vi "PmuAnalysis.vi"() -> ()   [LabVIEW 2018, in "Visualization.lvlib" / "VisualizeAnalysis.lvclass"]
uses:
  VisualizeAnalysis.lvclass
  VisualizeBase/VisualizeBase_class/SubVIs/VisualizationOptions.ctl
  <vilib>/Utility/miscctls.llb/LVRectTypeDef.ctl
  <vilib>/event_ctls.llb/usereventprio.ctl
  VisualizeBase/VisualizeBase_class/Requests/VisUserEventType.ctl
  <extravilib>/ChannelInstances/Tag-bool/Write With Abort.vi
  <extravilib>/ChannelInstances/Tag-bool/Read With Abort.vi
  <extravilib>/ChannelInstances/Tag-bool/Instantiate.vi
  <vilib>/Utility/error.llb/Error Cluster From Error Code.vi
  <extravilib>/ChannelInstances/Tag-bool/Endpoint.vi
  <vilib>/Utility/file.llb/Read From Spreadsheet File (DBL).vi
  <extravilib>/ChannelInstances/Tag-bool/EndpointRead.vi
  <vilib>/ErrorRing/Error Ring.xnode
  <userlib>/NIST/NISTErrorLib/NISTErrorLib.lvlib
  VisualizeBase/VisualizeBase_class/VisualizeBase.lvclass
  Analysis/AnalysisModule/AnalysisModule.lvlib
  Visualization.lvlib
  Sensor/VisualizeSensor.lvclass
  <extravilib>/ChannelInstances/Tag-bool.lvlib
  TestClass/Test.lvclass
  StatusAndLog/VisualizeStatus.lvclass
panel:
  in  "INIFilePath":path
  out "VisualizationProperties":T1={"PauseAtStartup"=TRUE, "LogData"=FALSE, "LaunchInSubPanel"=TRUE, "FPMonitor"=0, "FPWindowBounds"={"Left"=0, "Top"=0, "Right"=0, "Bottom"=0}, "MonitorBounds"={"Left"=0, "Top"=0, "Right"=0, "Bottom"=0}}
  in  "ModuleID":i32
  in  "btnClearTest":bool
  in  "btnReset":bool
  in  "btnPause":bool
  in  "btnOpen":bool
  in  "btnStop":bool
  in  "PluginName":string="Sensor.RoomAlert1"
  in  "Log Data":bool=TRUE
  out "Data from file":dbl[][](array[numeric])
  out "TVE":cluster{timestamp[], dbl[]}[](graph)
  out "FE":dbl(graph)=1.1347977483922023e-05
  out "ErrorArray":errorcluster[](array[cluster])
  out "RFE":dbl(graph)=-0.0019269131938461162
  out "Data real time":dbl[](array[numeric])
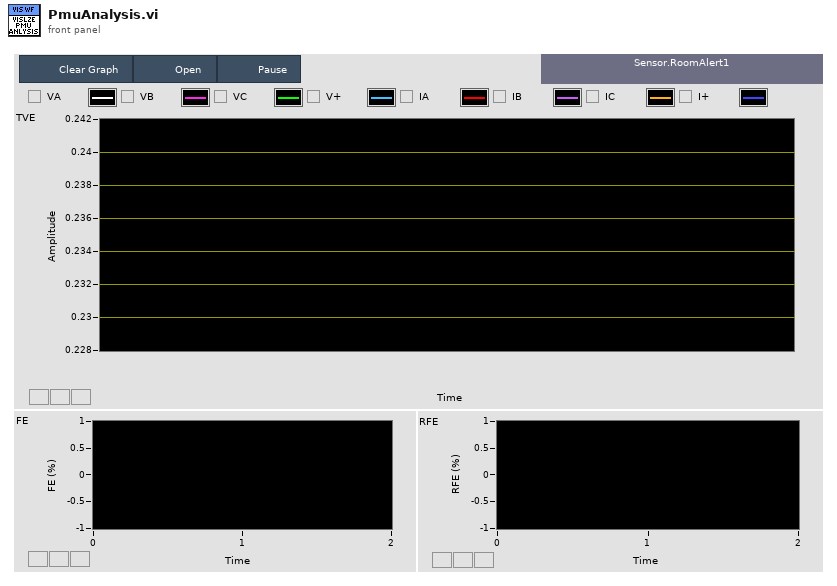
[diagram p1: front panel]
types:
  T1 = typedef "Visualization.lvlib/VisualizeBase.lvclass/VisualizationOptions.ctl" = cluster{"PauseAtStartup":bool, "LogData":bool, "LaunchInSubPanel":bool, "FPMonitor":u16, "FPWindowBounds":T2, "MonitorBounds":cluster{"Left":i16, "Top":i16, "Right":i16, "Bottom":i16}}
  T2 = typedef "LVRectTypeDef.ctl" = cluster{"Left":i16, "Top":i16, "Right":i16, "Bottom":i16}
  T3 = typedef "Visualization.lvlib/VisualizeBase.lvclass/VisRequestEvents.ctl" = cluster{"StopRequest":refnum<user-event>, "ResetRequest":refnum<user-event>, "FP Pop In or Out":refnum<user-event>}
  T4 = typedef "AnalysisModule.lvlib/clBroadcastEvents.ctl" = cluster{"DidInit":refnum<user-event>, "StatusUpdate":refnum<user-event>, "ErrorReport":refnum<user-event>, "DidStop":refnum<user-event>, "PathToINI":refnum<user-event>, "Config":refnum<user-event>, "ResultReport":refnum<user-event>, "FunctionClass":refnum<user-event>, "State":refnum<user-event>, "FunctionParams":refnum<user-event>, "Duration":refnum<user-event>}
  T5 = enum16{"open", "open or create", "create or replace", "create", "open (read-only)"}
  T6 = typedef "Visualization.lvlib/VisualizeBase.lvclass/VisUserEventType.ctl" = cluster{"BusIndex":i8, "Data":variant}
  T7 = typedef "usereventprio.ctl" = enum32{"high priority", "normal priority"}
  T8 = typedef "Tag-bool.lvlib/))Channel.ctl" = refnum<queue>
  T9 = typedef "sizeaction.ctl" = enum32{"Minimized", "Maximized", "Resized"}
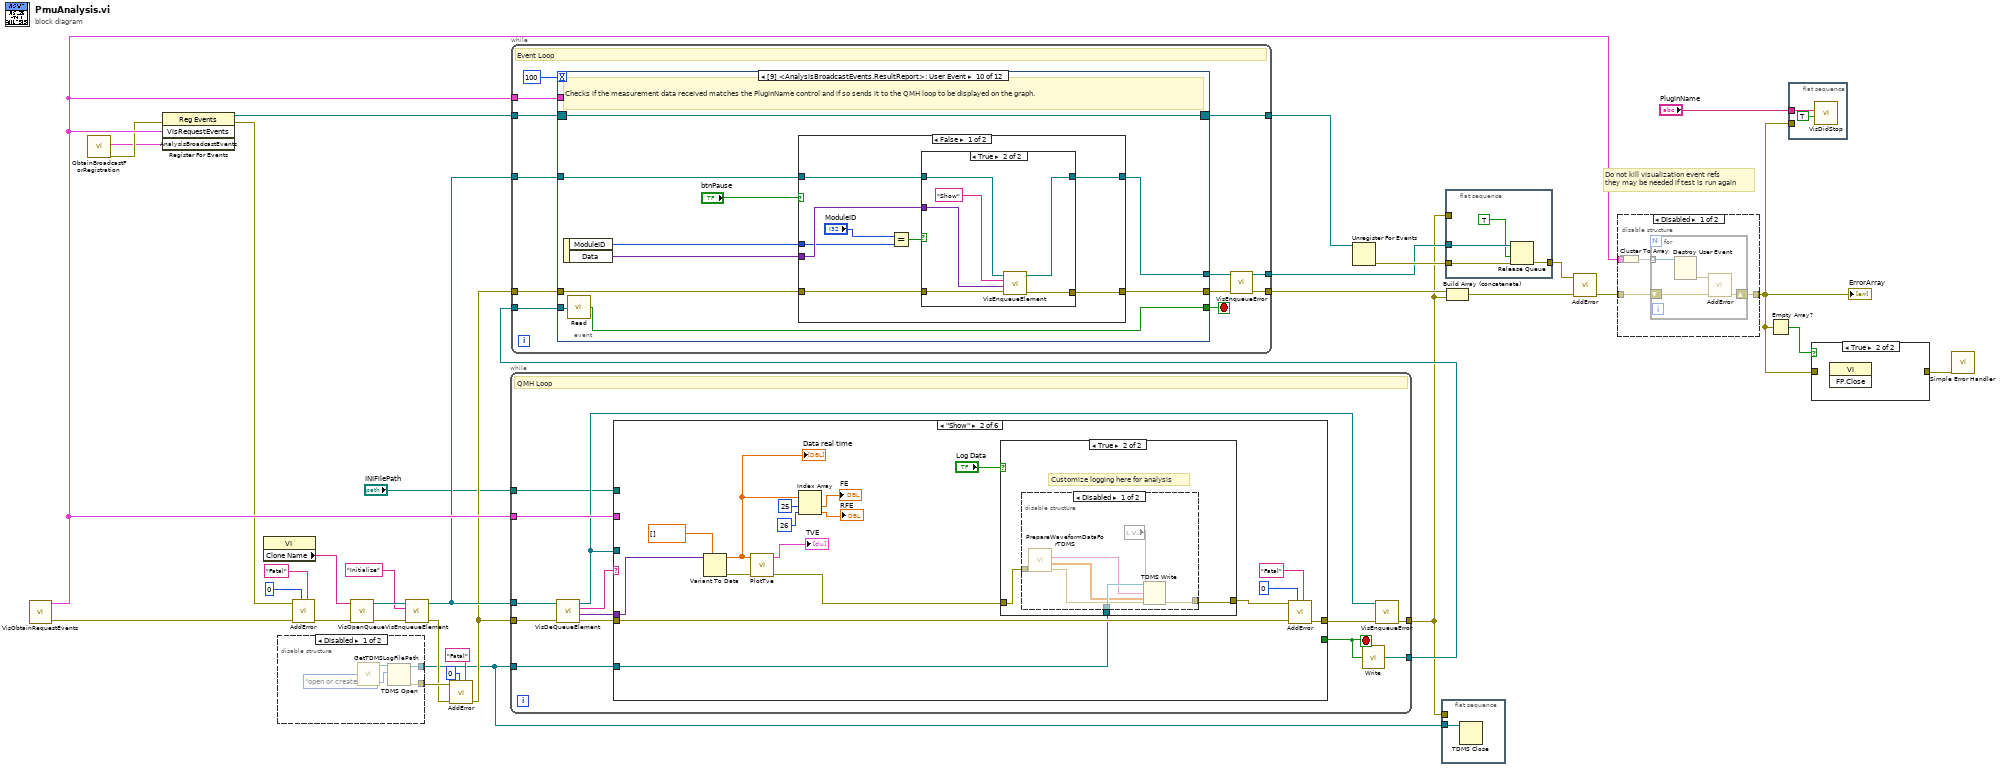
[diagram p0: block diagram]
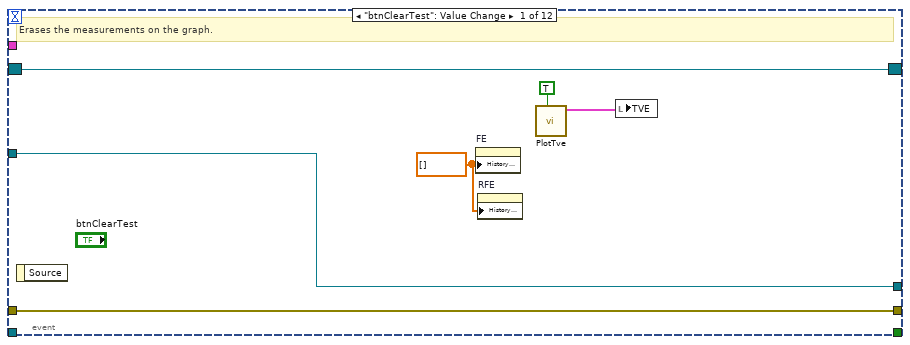
[diagram p4: hidden frame]
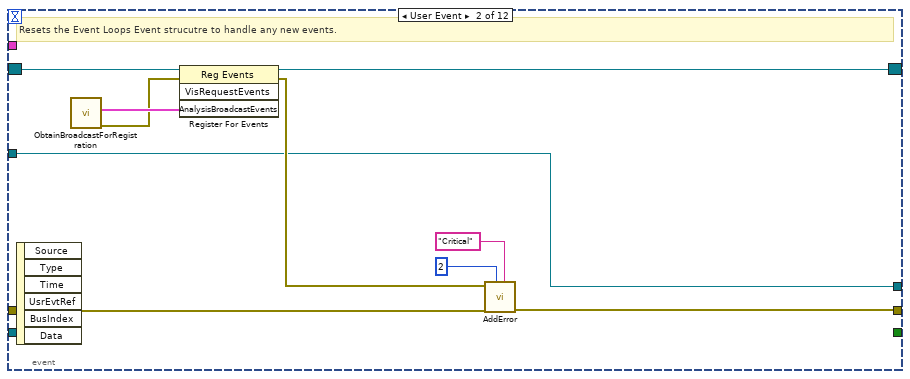
[diagram p5: hidden frame]
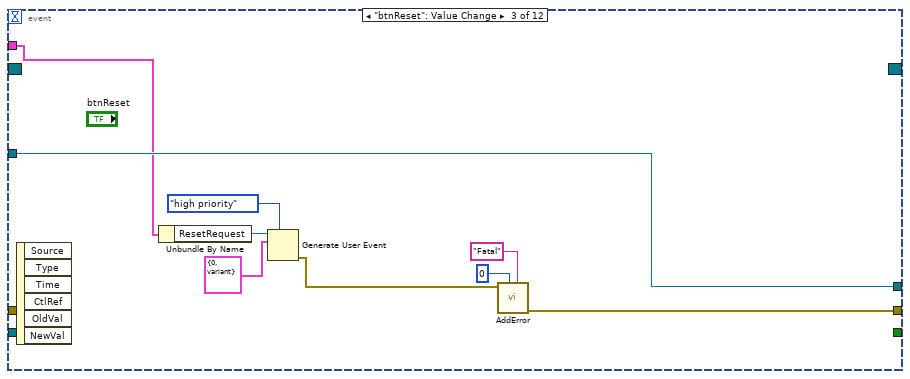
[diagram p6: hidden frame]
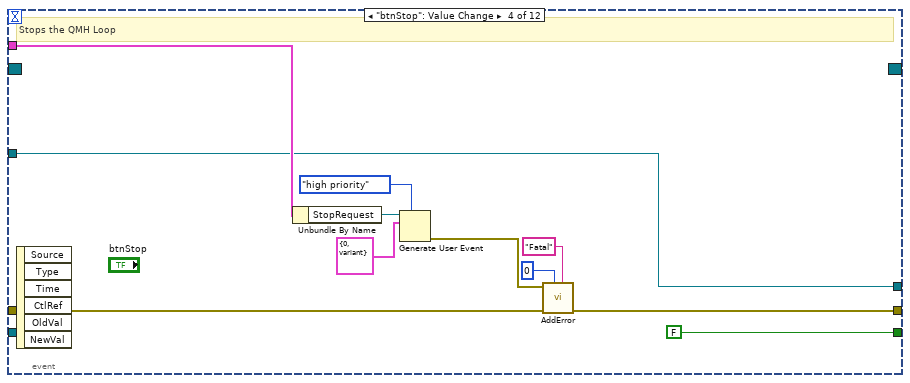
[diagram p7: hidden frame]
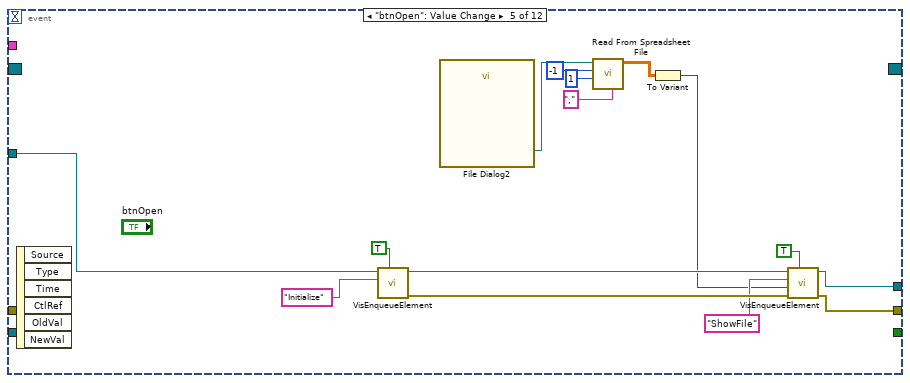
[diagram p8: hidden frame]
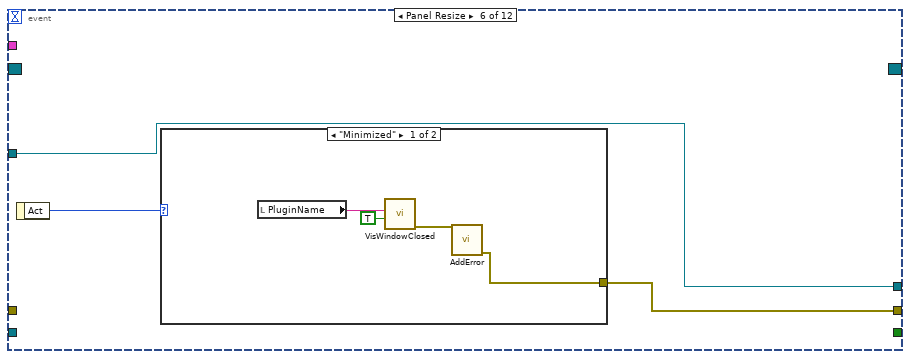
[diagram p9: hidden frame]
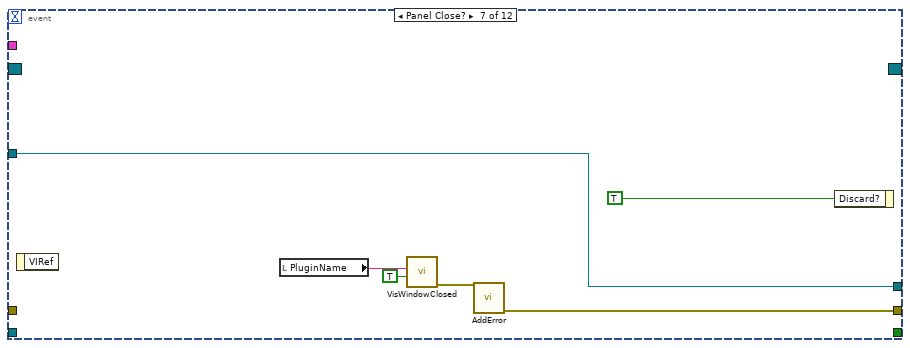
[diagram p11: hidden frame]
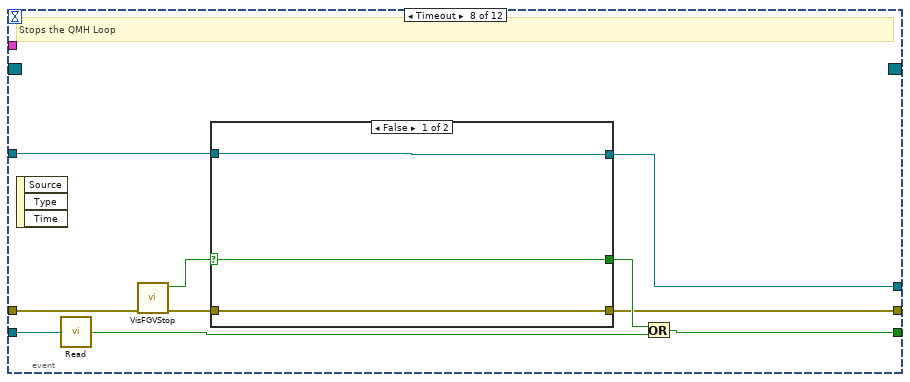
[diagram p12: hidden frame]
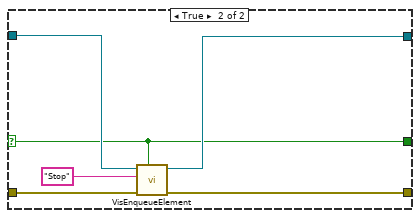
[diagram p13: hidden frame]
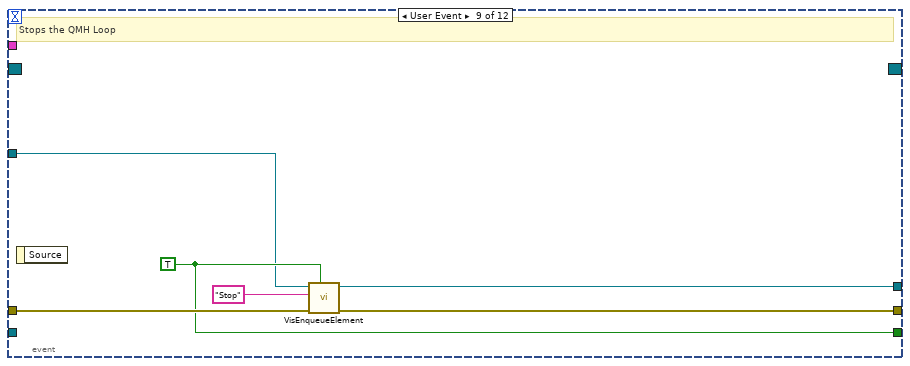
[diagram p14: hidden frame]
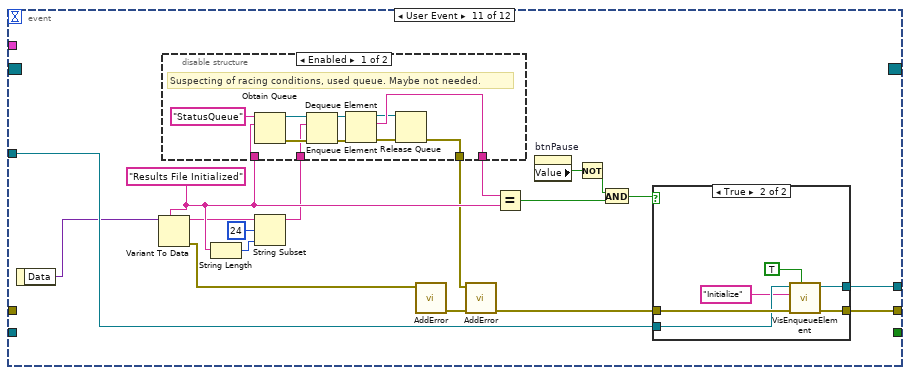
[diagram p17: hidden frame]
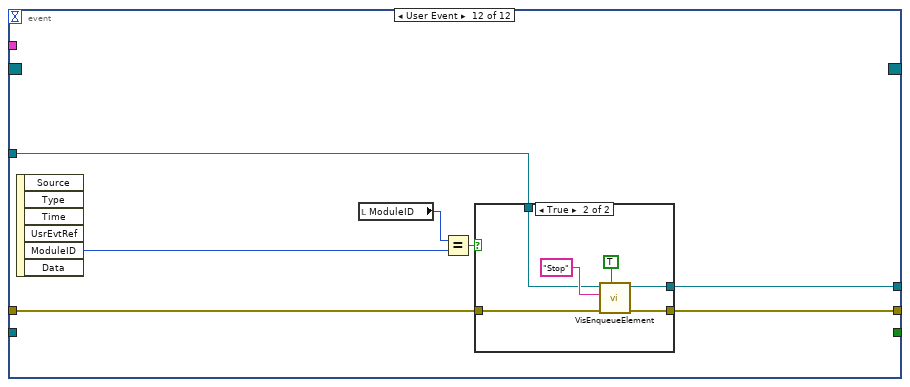
[diagram p20: hidden frame]
diagram:
  # "Do not kill visualization event refs\nthey may be needed if test is run again"
  n1 = call "VisObtainRequestEvents.vi"() -> ("Error"=w25:errorcluster[], "VisRequestEvents"=w27:T3)  [unwired: 10 in]
  n2 = call "ObtainBroadcastForRegistration.vi"() -> ("error out"=w5:errorcluster, "AnalysisBroadcastEvents"=w4:T4)  [unwired: 10 in]
  n3 = register-events(error in=w5, w27, w4) -> (reference out=w34:refnum<event-registration>, error out=w24:errorcluster)  [unwired: 1 in]
  n4 = property class="VI"() -> ("Clone Name"=w13:string)  [unwired: 2 in, 2 out]
  n5 = disable-structure shown="Disabled" {
    disable-tunnel: [w37 _] -> w10
    disable-tunnel: [w35 _] -> w7
    frame Disabled {
      n6 = call "GetTDMSLogFilePath.vi"() -> ("TDMS Log File Path"=w38:path)  [unwired: 11 in]
      n7 = TDMS Open(10:T5."open or create" ("operation (0:open)"), 11:w38) -> (0:w37:errorcluster, 3:w35:refnum<k34>)  [unwired: 5 in]
    }
    frame Enabled {
    }
  }
  n8 = call <userlib>:"AddError.vi"("Severity"="Fatal", "Priority"=u8 0, "ErrorArray In"=w25, "error in (no error)"=w24) -> ("ErrorArray Out"=w21:errorcluster[])  [unwired: 6 in, 1 out]
  n9 = call "VisOpenQueue.vi"("Error Array In"=w21, "QueueName"=w13) -> ("Error Array Out"=w19:errorcluster[], "queue out"=w20:refnum<queue>)  [unwired: 8 in]
  n10 = call "VisEnqueueElement.vi"("Error Array In"=w19, "Message"="Initialize", "queue in"=w20) -> ("Error Array Out"=w9:errorcluster[], "queue out"=w17:refnum<queue>)  [unwired: 7 in]
  n11 = call <userlib>:"AddError.vi"("Severity"="Fatal", "Priority"=u8 0, "ErrorArray In"=w9, "error in (no error)"=w10) -> ("ErrorArray Out"=w8:errorcluster[])  [unwired: 6 in, 1 out]
  n12 = while {
    tunnel: w8 -> [w45]
    tunnel: [w48] -> w6
    tunnel: w17 -> [w44]
    tunnel: w27 -> [w50]
    tunnel: [w41] -> w14
    tunnel: w7 -> [w40]
    tunnel: "INIFilePath" -> [w39]
    stop <- w51 stop-if-true
    # "QMH Loop"
    n13 = call "VisDeQueueElement.vi"("Error Array In"=w45, "Queue In"=w44) -> ("Error Array Out"=w43:errorcluster[], "Data"=w46:variant, "Message"=w47:string, "Queue Out"=w42:refnum<queue>)  [unwired: 6 in]
    n14 = case shown="\"Show\"" w47 {
      selector: w47 -> [_ _ _ w114 _ _]
      tunnel: w46 -> [_ w63 w89 _ w133 _]
      tunnel: w43 -> [w55 w76 _ w112 _ w162]
      tunnel: [w54 w77 _ w111 w123 w161] -> w49
      tunnel: [_ _ _ _ w129 TRUE] -> w51
      tunnel: w50 -> [_ _ _ _ w128 _]
      tunnel: w42 -> [_ _ _ _ w127 _]
      tunnel: w40 -> [_ w71 _ _ _ _]
      tunnel: w39 -> [w53 _ _ _ _ w160]
      frame "Initialize" {
        w60 = dbl[] [] ("History Data")
        (unwired) dbl[][] [] ("History Data")
        n15 = call "ApplyVisOptions.vi"("INIFilePath"=w53) -> ("error out"=w56:errorcluster, "VisualizationProperties"=→"VisualizationProperties":T1)  [unwired: 9 in]
        n16 = call <userlib>:"AddError.vi"("Severity"="Inform", "ErrorArray In"=w55, "error in (no error)"=w56) -> ("ErrorArray Out"=w54:errorcluster[])  [unwired: 7 in, 1 out]
        n17 = property on="FE" class="WFChart (strict)"("History Data"=w60) -> ()  [unwired: 2 in, 2 out]
        n18 = property on="RFE" class="WFChart (strict)"("History Data"=w60) -> ()  [unwired: 2 in, 2 out]
        n19 = call "PlotTve.vi"("Clear? (f)"=TRUE) -> ("TVE"=w58:cluster{timestamp[], dbl[]}[])  [unwired: 9 in, 1 out]
        n20 = property on="TVE" class="XYGraph (strict)"("Value"=w58) -> ()  [unwired: 2 in, 2 out]
      }
      frame "Show" {
        n21 = Variant To Data(type=dbl[] [], Variant=w63) -> (data=w68:dbl[], error out=w61:errorcluster)  [unwired: 1 in]
        "Data real time" <- w68
        n22 = call "PlotTve.vi"("error in (no error)"=w61, "Data real time"=w68) -> ("error out"=w62:errorcluster, "TVE"=→"TVE":cluster{timestamp[], dbl[]}[])  [unwired: 8 in]
        n23 = Index Array(array=w68, index #1=25 ("index"), index #2=26 ("index")) -> (element #1=→"FE":dbl, element #2=→"RFE":dbl)
        n24 = case shown="True" "Log Data" {
          tunnel: w62 -> [w78 w80]
          tunnel: [w78 w81] -> w73
          tunnel: w71 -> [_ w79]
          frame False {
          }
          frame True {
            # "Customize logging here for analysis"
            n25 = disable-structure shown="Disabled" {
              disable-tunnel: [w88 _] -> w81
              disable-tunnel: w80 -> [w87 _]
              disable-tunnel: w79 -> [w85 _]
              frame Disabled {
                n26 = call "PrepareWaveformDataForTDMS.vi"("error in (no error)"=w87) -> ("error out"=w84:errorcluster, "Measurement Data"=w82:dbl[][], "Channel Names"=w83:string[])  [unwired: 8 in]
                n27 = local read item#-1() -> (w86)
                n28 = TDMS Write(0:w85, 5:w86, 7:w83, 9:w82, 11:w84) -> (15:w88:errorcluster)  [unwired: 1 in, 3 out]
              }
              frame Enabled {
              }
            }
          }
        }
        n29 = call <userlib>:"AddError.vi"("Severity"="Fatal" ("String"), "Priority"=u8 0, "ErrorArray In"=w76, "error in (no error)"=w73) -> ("ErrorArray Out"=w77:errorcluster[])  [unwired: 6 in, 1 out]
      }
      frame "ShowFile" {
        n30 = Variant To Data(type=dbl[][] [], Variant=w89) -> (data=w102:dbl[][])  [unwired: 1 in, 1 out]
        "Data from file" <- w102
        n31 = Index Array(array=w102, index (col) #1=1 ("disabled index (col)"), index (col) #2=4 ("index (col)"), index (col) #3=7 ("index (col)"), index (col) #4=10 ("index (col)")) -> (element #1=w98:dbl[], element #2=w99:dbl[], element #3=w100:dbl[], element #4=w105:dbl[])  [unwired: 4 in]
        n32 = Index Array(array=w102, index (col) #1=25 ("disabled index (col)"), index (col) #2=26 ("index (col)")) -> (element #1=w103:dbl[], element #2=w104:dbl[])  [unwired: 2 in]
        n33 = Array Size(array=w105) -> (size(s)=w106:i32)
        n34 = Initialize Array(1.0 ("element"), w106) -> (w107:dbl[])
        n35 = property on="FE" class="WFChart (strict)"("History Data"=w103) -> ()  [unwired: 2 in, 2 out]
        n36 = Build Array(w98, w99, w100, w105, w107) -> (w101:dbl[][])
        n37 = property on="RFE" class="WFChart (strict)"("History Data"=w104) -> ()  [unwired: 2 in, 2 out]
        n38 = Transpose 2D Array(2D array=w101) -> ()  [unwired: 1 out]
      }
      frame Default {
        n39 = xnode "Error Ring"("parameter 0"=w114) -> ("error out"=w113:errorcluster)
        n40 = call <userlib>:"AddError.vi"("Severity"="Inform" ("String"), "Priority"=u8 5, "ErrorArray In"=w112, "error in (no error)"=w113) -> ("ErrorArray Out"=w111:errorcluster[], "error out"=w110:errorcluster)  [unwired: 6 in]
        n41 = call <vilib>:"Clear Errors.vi"("error in (no error)"=w110) -> ()  [unwired: 5 in, 2 out]
      }
      frame "Error" {
        n42 = Variant To Data(type=errorcluster[] [], Variant=w133) -> (data=w131:errorcluster[], error out=w122:errorcluster)  [unwired: 1 in]
        n43 = call <userlib>:"ParseErrors.vi"("ErrorArray"=w131) -> ("ErrorArray"=w130:errorcluster[])  [unwired: 8 in, 2 out]
        n44 = for {
          tunnel: w130 -> [w144] mode=indexing
          tunnel: [w138] -> w124 mode=concatenating
          tunnel: [w136] -> w129
          tunnel: w128 -> [w135]
          tunnel: w127 -> [w134]
          stop <- w136 stop-if-true
          n45 = call <userlib>:"GeneralHandler.vi"("error in (no error)"=w144) -> ("Severity"=w137:string, "Stop"=w141:bool, "Abort"=w142:bool, "Continue"=w143:bool)  [unwired: 6 in, 1 out]
          n46 = Build Array(w143, w142, w141) -> (w140:bool[])
          n47 = Boolean Array To Number(Boolean array=w140) -> (number=w139:u32)
          n48 = case shown="4" w139 {
            tunnel: [_ _ w149 w158] -> w138
            tunnel: w137 -> [_ _ _ w151]
            tunnel: [_ _ _ w153] -> w136
            tunnel: w135 -> [_ _ _ w152]
            tunnel: w134 -> [_ _ w145 _]
            frame 0, Default {
              # "No Dialog"
            }
            frame 1 {
              # "Continue"
            }
            frame 2 {
              # "Abort, Flush Queue"
              n49 = Flush Queue(queue=w145) -> (error out=w148:errorcluster)  [unwired: 1 in, 2 out]
              n50 = call <userlib>:"AddError.vi"("Severity"="Critical" ("String"), "Priority"=u8 1, "error in (no error)"=w148) -> ("ErrorArray Out"=w149:errorcluster[])  [unwired: 7 in, 1 out]
            }
            frame 4 {
              # "Stop"
              n51 = Unbundle By Name(w152) -> ("StopRequest"=w159:refnum<user-event>)
              n52 = Equal?(x=w151, y="Fatal" ("x")) -> (x = y?=w153:bool)
              n53 = Generate User Event(priority (normal)=usereventprio."high priority", user event=w159, event data cluster=T6 {"BusIndex"=0, "Data"=variant} ("event data")) -> (error out=w157:errorcluster)  [unwired: 1 in, 1 out]
              n54 = call <userlib>:"AddError.vi"("error in (no error)"=w157) -> ("ErrorArray Out"=w158:errorcluster[], "error out"=w154:errorcluster)  [unwired: 9 in]
              n55 = call <vilib>:"Clear Errors.vi"("error in (no error)"=w154) -> ()  [unwired: 5 in, 2 out]
            }
          }
        }
        n56 = call <userlib>:"AddError.vi"("Severity"="Critical", "Priority"=u8 2, "ErrorArray In"=w124, "error in (no error)"=w122) -> ("ErrorArray Out"=w123:errorcluster[])  [unwired: 6 in, 1 out]
      }
      frame "Stop" {
        n57 = local read "VisualizationProperties"() -> (w163:T1)
        n58 = call "WriteVisOptionsToINIFile.vi"("Visualization Options"=w163, "INIFilePath"=w160) -> ("error out"=w165:errorcluster)  [unwired: 8 in, 1 out]
        n59 = call <userlib>:"AddError.vi"("Severity"="Inform", "ErrorArray In"=w162, "error in (no error)"=w165) -> ("ErrorArray Out"=w161:errorcluster[])  [unwired: 7 in, 1 out]
      }
    }
    n60 = call <extravilib>:"Write.vi"("element"=w51) -> ("channel"=w41:T8)  [unwired: 1 out]
    n61 = call "VisEnqueueError.vi"("Error Array In"=w49, "Queue in"=w42) -> ("Error Array Out"=w48:errorcluster[])  [unwired: 8 in, 1 out]
  }
  n62 = while {
    tunnel: w34 -> [w178]
    tunnel: [w172] -> w32
    tunnel: [w176] -> w33
    tunnel: w27 -> [w175]
    tunnel: w8 -> [w174]
    tunnel: w17 -> [w173]
    tunnel: [w169] -> w16
    tunnel: w14 -> [w167]
    stop <- w177 stop-if-true
    # "Event Loop"
    n63 = event shown="[9] <AnalysisBroadcastEvents.ResultReport>: User Event" {
      selector: w178 -> [w183 w194 _ _ _ _ _ _ _ w273 _ _]
      dyn-events: [w183 w193 _ _ _ _ _ _ _ w273 _ _] -> w176
      timeout: 100 -> [_ _ _ _ _ _ _ _ _ _ _ _]
      tunnel: [_ _ _ FALSE ("Priority? (F)") _ _ _ w243 w264 w270 _ _] -> w177
      tunnel: [w184 w191 w197 w207 w216 w231 w237 w245 w266 w275 w298 w338] -> w171
      tunnel: w175 -> [_ _ w195 w206 _ _ _ _ _ _ _ _]
      tunnel: w174 -> [w184 w192 _ w214 _ _ _ w248 w267 w276 _ w336]
      tunnel: w173 -> [w182 w187 w196 w204 w224 w230 w241 w247 w262 w277 w300 w337]
      tunnel: [w182 w187 w196 w204 w215 w230 w241 w246 w265 w274 w297 w339] -> w170
      tunnel: w167 -> [_ _ _ _ _ _ _ w252 _ w271 _ _]
      event "btnClearTest": Value Change {
        w181 = dbl[] [] ("History Data")
        # "Erases the measurements on the graph."
        n64 = event-data() -> ()  [unwired: 1 in, 1 out]
        n65 = property on="FE" class="WFChart (strict)"("History Data"=w181) -> ()  [unwired: 2 in, 2 out]
        n66 = property on="RFE" class="WFChart (strict)"("History Data"=w181) -> ()  [unwired: 2 in, 2 out]
        n67 = call "PlotTve.vi"("Clear? (f)"=TRUE) -> ("TVE"=w180:cluster{timestamp[], dbl[]}[])  [unwired: 9 in, 1 out]
        n68 = local write "TVE"(w180) -> ()
      }
      event User Event {
        # "Resets the Event Loops Event strucutre to handle any new events."
        n69 = event-data() -> ()  [unwired: 1 in, 6 out]
        n70 = call "ObtainBroadcastForRegistration.vi"() -> ("error out"=w185:errorcluster, "AnalysisBroadcastEvents"=w186:T4)  [unwired: 10 in]
        n71 = register-events(reference=w194, error in=w185, w186) -> (reference out=w193:refnum<event-registration>, error out=w188:errorcluster)  [unwired: 1 in]
        n72 = call <userlib>:"AddError.vi"("Severity"="Critical", "Priority"=u8 2, "ErrorArray In"=w192, "error in (no error)"=w188) -> ("ErrorArray Out"=w191:errorcluster[])  [unwired: 6 in, 1 out]
      }
      event "btnReset": Value Change {
        n73 = event-data() -> ()  [unwired: 1 in, 6 out]
        n74 = Unbundle By Name(w195) -> ("ResetRequest"=w203:refnum<user-event>)
        n75 = Generate User Event(priority (normal)=usereventprio."high priority", user event=w203, event data cluster=T6 {"BusIndex"=0, "Data"=variant} ("event data")) -> (error out=w200:errorcluster)  [unwired: 1 in, 1 out]
        n76 = call <userlib>:"AddError.vi"("Severity"="Fatal", "Priority"=u8 0, "error in (no error)"=w200) -> ("ErrorArray Out"=w197:errorcluster[])  [unwired: 7 in, 1 out]
      }
      event "btnStop": Value Change {
        # "Stops the QMH Loop"
        n77 = event-data() -> ()  [unwired: 1 in, 6 out]
        n78 = Unbundle By Name(w206) -> ("StopRequest"=w212:refnum<user-event>)
        n79 = Generate User Event(priority (normal)=usereventprio."high priority", user event=w212, event data cluster=T6 {"BusIndex"=0, "Data"=variant} ("event data")) -> (error out=w213:errorcluster)  [unwired: 1 in, 1 out]
        n80 = call <userlib>:"AddError.vi"("Severity"="Fatal" ("String"), "Priority"=u8 0, "ErrorArray In"=w214, "error in (no error)"=w213) -> ("ErrorArray Out"=w207:errorcluster[])  [unwired: 6 in, 1 out]
      }
      event "btnOpen": Value Change {
        n81 = event-data() -> ()  [unwired: 1 in, 6 out]
        n82 = call "VisEnqueueElement.vi"("Priority? (F)"=TRUE, "Message"="Initialize", "queue in"=w224) -> ("Error Array Out"=w220:errorcluster[], "queue out"=w218:refnum<queue>)  [unwired: 7 in]
        n83 = call "File Dialog2"() -> ("selected path"=w225:path)  [unwired: 12 in, 3 out]
        n84 = call-poly <vilib>:"Read From Spreadsheet File.vi"("delimiter (\\t)"="," ("delimiter (\\t)"), "start of read offset (chars.:0)"=1, "number of rows (all:-1)"=-1, "file path (dialog if empty)"=w225) -> ("all rows"=w227:dbl[][])  [unwired: 3 in, 4 out]
        n85 = To Variant(anything=w227) -> (Variant=w217:variant)
        n86 = call "VisEnqueueElement.vi"("Priority? (F)"=TRUE, "Error Array In"=w220, "Data"=w217, "Message"="ShowFile", "queue in"=w218) -> ("Error Array Out"=w216:errorcluster[], "queue out"=w215:refnum<queue>)  [unwired: 5 in]
      }
      event Panel Resize {
        n87 = event-data() -> ("Act"=w232:T9)  [unwired: 1 in]
        n88 = case shown="\"Minimized\"" w232 {
          tunnel: [w233 _] -> w231
          frame "Minimized" {
            n89 = local read "PluginName"() -> (w235:string)
            n90 = call "VisWindowClosed.vi"("Window Closed?"=TRUE ("Window Minimized or Clozed?"), "Module Name"=w235) -> ("error out"=w236:errorcluster)  [unwired: 9 in]
            n91 = call <userlib>:"AddError.vi"("error in (no error)"=w236) -> ("ErrorArray Out"=w233:errorcluster[])  [unwired: 9 in, 1 out]
          }
          frame "Maximized", Default {
          }
        }
      }
      event Panel Close? {
        n92 = event-data() -> ()  [unwired: 1 in, 1 out]
        n93 = local read "PluginName"() -> (w238:string)
        n94 = call "VisWindowClosed.vi"("Window Closed?"=TRUE ("Window Minimized or Clozed?"), "Module Name"=w238) -> ("error out"=w240:errorcluster)  [unwired: 9 in]
        n95 = call <userlib>:"AddError.vi"("error in (no error)"=w240) -> ("ErrorArray Out"=w237:errorcluster[])  [unwired: 9 in, 1 out]
        n96 = event-data("Discard?"=TRUE) -> ()  [unwired: 1 in, 1 out]
      }
      event Timeout {
        # "Stops the QMH Loop"
        n97 = event-data() -> ()  [unwired: 1 in, 3 out]
        n98 = call <extravilib>:"Read.vi"("channel"=w252) -> ("element"=w244:bool)  [unwired: 1 in, 1 out]
        n99 = call "VisFGVStop.vi"("Error In"=w248) -> ("Error Out"=w250:errorcluster[], "Value"=w251:bool)  [unwired: 9 in]
        n100 = case shown="False" w251 {
          selector: w251 -> [w253 w256]
          tunnel: [w255 w259] -> w245
          tunnel: w250 -> [w255 w260]
          tunnel: w247 -> [w254 w258]
          tunnel: [w254 w257] -> w246
          tunnel: [w253 w256] -> w249
          frame False {
          }
          frame True {
            n101 = call "VisEnqueueElement.vi"("Priority? (F)"=w256, "Error Array In"=w260, "Message"="Stop", "queue in"=w258) -> ("Error Array Out"=w259:errorcluster[], "queue out"=w257:refnum<queue>)  [unwired: 6 in]
          }
        }
        n102 = Or(x=w249, y=w244) -> (x .or. y?=w243:bool)
      }
      event User Event {
        w264 = TRUE ("Priority? (F)")
        # "Stops the QMH Loop"
        n103 = event-data() -> ()  [unwired: 1 in, 1 out]
        n104 = call "VisEnqueueElement.vi"("Priority? (F)"=w264, "Error Array In"=w267, "Message"="Stop", "queue in"=w262) -> ("Error Array Out"=w266:errorcluster[], "queue out"=w265:refnum<queue>)  [unwired: 6 in]
      }
      event User Event {
        # "Checks if the measurement data received matches the PluginName control and if so sends it to the QMH loop to be displayed on the graph."
        n105 = event-data() -> ("ModuleID"=w268:i32, "Data"=w272:variant)  [unwired: 1 in]
        n106 = call <extravilib>:"Read.vi"("channel"=w271) -> ("element"=w270:bool)  [unwired: 1 in, 1 out]
        n107 = case shown="False" "btnPause" {
          tunnel: w277 -> [w285 w295]
          tunnel: w276 -> [w284 w294]
          tunnel: [w278 w294] -> w275
          tunnel: [w283 w295] -> w274
          tunnel: w272 -> [w282 _]
          tunnel: w268 -> [w281 _]
          frame False {
            n108 = Equal?(x="ModuleID", y=w281) -> (x = y?=w280:bool)
            n109 = case shown="True" w280 {
              tunnel: [w286 w292] -> w278
              tunnel: w285 -> [w287 w291]
              tunnel: w284 -> [w286 w293]
              tunnel: [w287 w289] -> w283
              tunnel: w282 -> [_ w290]
              frame False {
              }
              frame True {
                n110 = call "VisEnqueueElement.vi"("Error Array In"=w293, "Data"=w290, "Message"="Show", "queue in"=w291) -> ("Error Array Out"=w292:errorcluster[], "queue out"=w289:refnum<queue>)  [unwired: 6 in]
              }
            }
          }
          frame True {
          }
        }
      }
      event User Event {
        w310 = "Results File Initialized" ("Status")
        n111 = event-data() -> ("Data"=w299:variant)  [unwired: 1 in]
        n112 = Variant To Data(type=w310, Variant=w299) -> (data=w302:string, error out=w305:errorcluster)  [unwired: 1 in]
        n113 = String Length(string=w310) -> (length=w309:i32)
        n114 = String Subset(string=w302, offset (0)=24, length (rest)=w309) -> (substring=w307:string)
        n115 = disable-structure shown="Enabled" {
          disable-tunnel: [w317 w325] -> w303
          disable-tunnel: [w314 _] -> w306
          disable-tunnel: w307 -> [w319 w325]
          disable-tunnel: w310 -> [w318 _]
          frame Enabled {
            # "Suspecting of racing conditions, used queue. Maybe not needed."
            n116 = Obtain Queue(name (unnamed)="StatusQueue", element data type=w318) -> (queue out=w323:refnum<queue>, error out=w321:errorcluster)  [unwired: 3 in, 1 out]
            n117 = Enqueue Element(queue=w323, element=w319, error in (no error)=w321) -> (queue out=w322:refnum<queue>, error out=w320:errorcluster)  [unwired: 1 in, 1 out]
            n118 = Dequeue Element(queue=w322, error in (no error)=w320) -> (queue out=w316:refnum<queue>, element=w317:string, error out=w315:errorcluster)  [unwired: 1 in, 1 out]
            n119 = Release Queue(queue=w316, error in (no error)=w315) -> (error out=w314:errorcluster)  [unwired: 1 in, 2 out]
          }
          frame Disabled {
          }
        }
        n120 = call <userlib>:"AddError.vi"("error in (no error)"=w305) -> ("ErrorArray Out"=w304:errorcluster[])  [unwired: 9 in, 1 out]
        n121 = call <userlib>:"AddError.vi"("ErrorArray In"=w304, "error in (no error)"=w306) -> ("ErrorArray Out"=w301:errorcluster[])  [unwired: 8 in, 1 out]
        n122 = Equal?(x=w303, y=w310) -> (x = y?=w311:bool)
        n123 = property on="btnPause" class="Bool (strict)"() -> ("Value"=w312:bool)  [unwired: 2 in, 2 out]
        n124 = Not(x=w312) -> (.not. x?=w313:bool)
        n125 = And(x=w313, y=w311) -> (x .and. y?=w296:bool)
        n126 = case shown="True" w296 {
          tunnel: [w327 w332] -> w298
          tunnel: w301 -> [w327 w333]
          tunnel: w300 -> [w326 w331]
          tunnel: [w326 w328] -> w297
          frame False {
          }
          frame True {
            n127 = call "VisEnqueueElement.vi"("Priority? (F)"=TRUE, "Error Array In"=w333, "Message"="Initialize", "queue in"=w331) -> ("Error Array Out"=w332:errorcluster[], "queue out"=w328:refnum<queue>)  [unwired: 6 in]
          }
        }
      }
      event User Event {
        n128 = event-data() -> ("ModuleID"=w334:i32)  [unwired: 1 in, 5 out]
        n129 = local read "ModuleID"() -> (w335:i32)
        n130 = Equal?(x=w335, y=w334) -> (x = y?=w340:bool)
        n131 = case shown="True" w340 {
          tunnel: [w341 w346] -> w338
          tunnel: [w342 w345] -> w339
          tunnel: w337 -> [w342 w344]
          tunnel: w336 -> [w341 w343]
          frame False {
          }
          frame True {
            n132 = call "VisEnqueueElement.vi"("Priority? (F)"=TRUE, "Error Array In"=w343, "Message"="Stop", "queue in"=w344) -> ("Error Array Out"=w346:errorcluster[], "queue out"=w345:refnum<queue>)  [unwired: 6 in]
          }
        }
      }
    }
    n133 = call "VisEnqueueError.vi"("Error Array In"=w171, "Queue in"=w170) -> ("Error Array Out"=w172:errorcluster[], "Queue out"=w169:refnum<queue>)  [unwired: 8 in]
  }
  n134 = Unregister For Events(event registration refnum=w33) -> (error out=w31:errorcluster)  [unwired: 1 in]
  n135 = flat-sequence {
    tunnel: w7 -> [w349]
    tunnel: w6 -> [_]
    frame #0 {
      n136 = TDMS Close(11:w349) -> ()  [unwired: 1 in, 2 out]
    }
  }
  n137 = flat-sequence {
    tunnel: w31 -> [w353]
    tunnel: [w352] -> w29
    tunnel: w16 -> [w351]
    tunnel: w6 -> [_]
    frame #0 {
      n138 = Release Queue(queue=w351, force destroy? (F)=TRUE, error in (no error)=w353) -> (error out=w352:errorcluster)  [unwired: 2 out]
    }
  }
  n139 = Build Array (concatenate)(w32, w6) -> (w30:errorcluster[])
  n140 = call <userlib>:"AddError.vi"("ErrorArray In"=w30, "error in (no error)"=w29) -> ("ErrorArray Out"=w28:errorcluster[])  [unwired: 8 in, 1 out]
  n141 = disable-structure shown="Disabled" {
    disable-tunnel: w28 -> [w356 w362]
    disable-tunnel: w27 -> [w355 _]
    disable-tunnel: [w354 w362] -> w1
    frame Disabled {
      n142 = Cluster To Array(cluster=w355) -> (array=w357:refnum<user-event>[])
      n143 = for {
        tunnel: w357 -> [w361] mode=indexing
        shift-right: [w360] -> w354
        shift-left: w356 -> [w359]
        n144 = Destroy User Event(user event=w361) -> (error out=w358:errorcluster)  [unwired: 1 in]
        n145 = call <userlib>:"AddError.vi"("ErrorArray In"=w359, "error in (no error)"=w358) -> ("ErrorArray Out"=w360:errorcluster[])  [unwired: 8 in, 1 out]
      }
    }
    frame Enabled {
    }
  }
  "ErrorArray" <- w1
  n146 = Empty Array?(array=w1) -> (empty?=w26:bool)
  n147 = flat-sequence {
    tunnel: "PluginName" -> [w364]
    tunnel: w1 -> [_]
    frame #0 {
      n148 = call "VisDidStop.vi"("DidStop?"=TRUE, "Module Name"=w364) -> ()  [unwired: 9 in, 1 out]
    }
  }
  n149 = case shown="True" w26 {
    tunnel: [w365 _] -> w15
    tunnel: w1 -> [w366 _]
    frame False {
      n150 = Merge Errors(w366) -> (w365:errorcluster)
    }
    frame True {
      n151 = invoke class="VI" method="FP.Close"() -> ()  [unwired: 3 in, 3 out]
    }
  }
  n152 = call <vilib>:"Simple Error Handler.vi"("error in (no error)"=w15) -> ()  [unwired: 4 in, 5 out]
